vi "GV_Legend_DrawMove.vi"(2 "Legend":T1, 5 "Select":bool, 8 "Origin":cluster{"x":i16, "y":i16}) -> (7 "Image":picture)   [LabVIEW 2020, in "Sgraph_lib_V1.lvlib" / "Gviewer.lvclass"]
doc: "Andre Koelewijn, 25 April 2021,\n\nDraw arrows around the Legend to indicate the 'Legend-Move' grip.\nThe move action is then to be initiated by pressing the mouse button or the (s)elect button."
uses:
  Gviewer.lvclass
  controls/LegendSet.ctl
  <vilib>/Utility/miscctls.llb/LVPositionTypeDef.ctl
  <vilib>/Utility/miscctls.llb/LVBoundsTypeDef.ctl
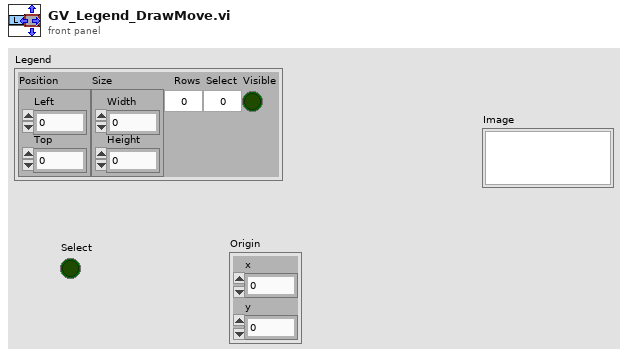
[diagram p1: front panel]
types:
  T1 = typedef "Sgraph_lib_V1.lvlib/Gviewer.lvclass/LegendSet.ctl" = cluster{"Position":T2, "Size":T3, "Rows":u32, "Select":i32, "Visible":bool}
  T2 = typedef "LVPositionTypeDef.ctl" = cluster{"Left":i32, "Top":i32}
  T3 = typedef "LVBoundsTypeDef.ctl" = cluster{"Width":u32, "Height":u32}
  T4 = cluster{"Width":u16, "Style":enum32{"Solid", "Dash", "Dot", "DashDot", "DashDotDot"}}
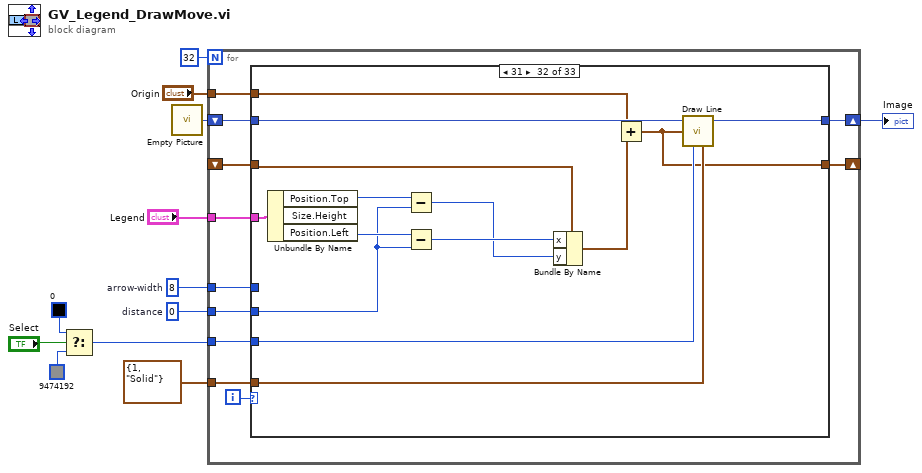
[diagram p0: block diagram]
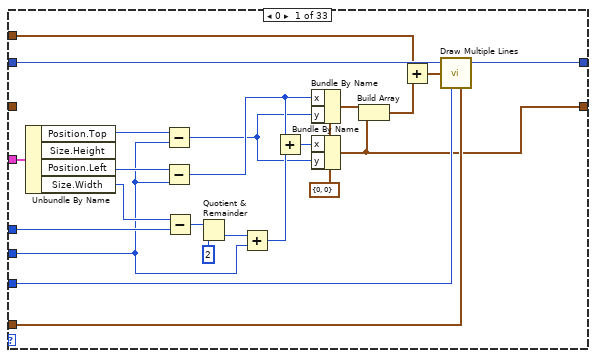
[diagram p2: hidden frame]
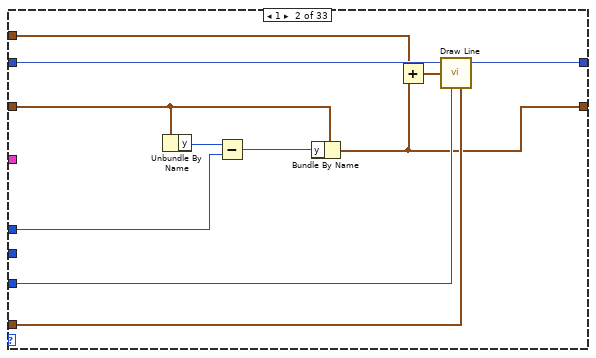
[diagram p3: hidden frame]
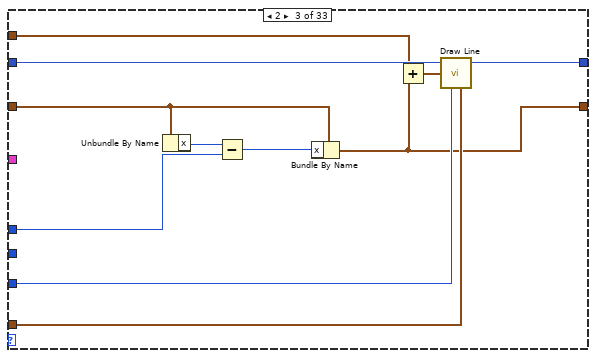
[diagram p4: hidden frame]
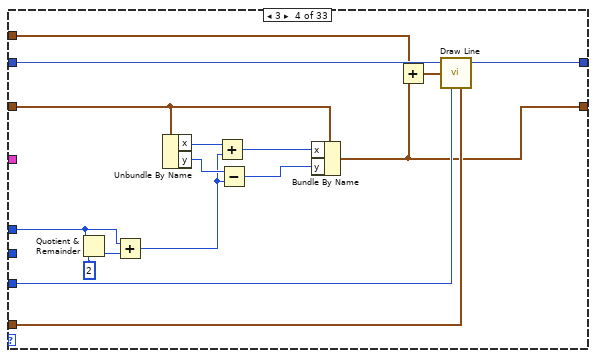
[diagram p5: hidden frame]
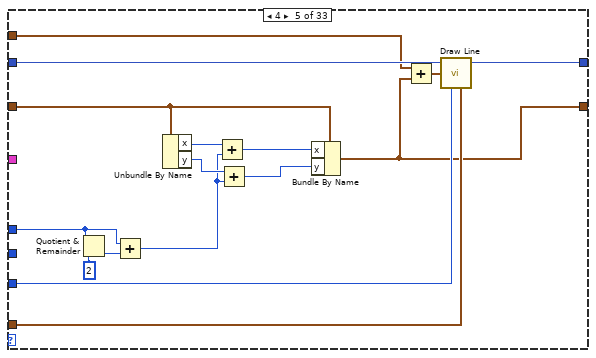
[diagram p6: hidden frame]
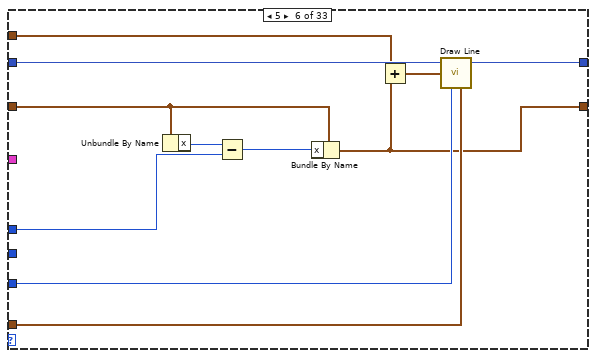
[diagram p7: hidden frame]
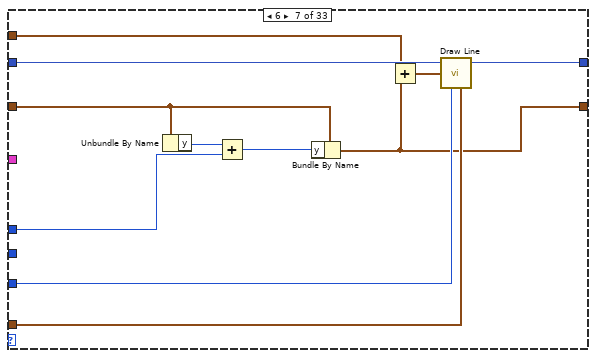
[diagram p8: hidden frame]
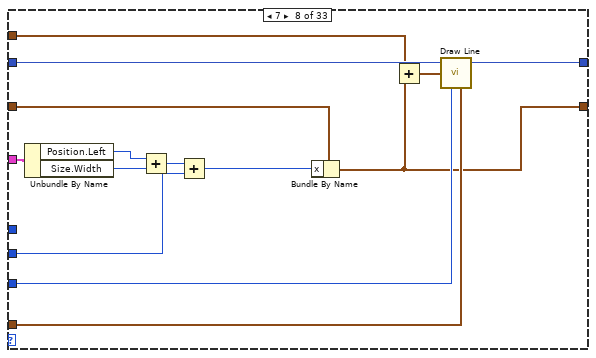
[diagram p9: hidden frame]
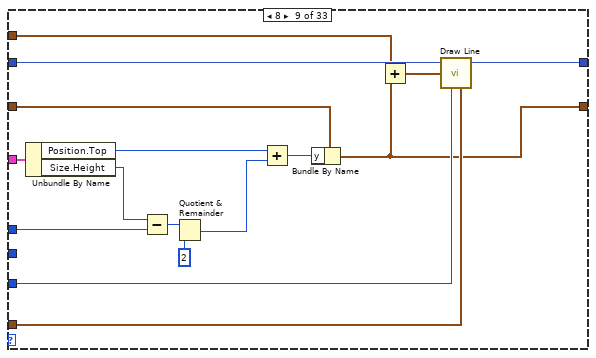
[diagram p10: hidden frame]
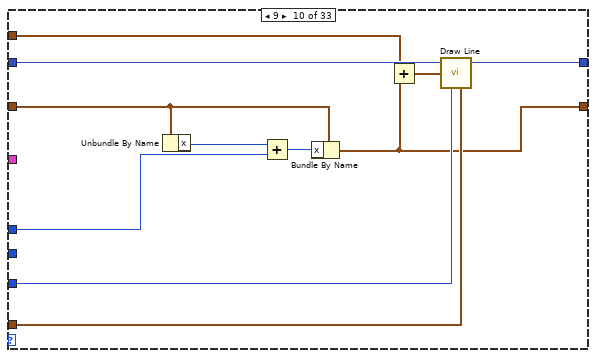
[diagram p11: hidden frame]
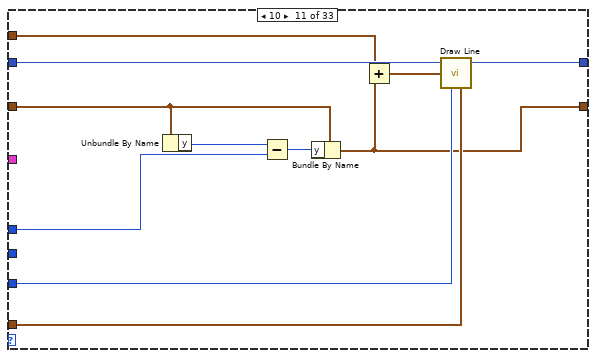
[diagram p12: hidden frame]
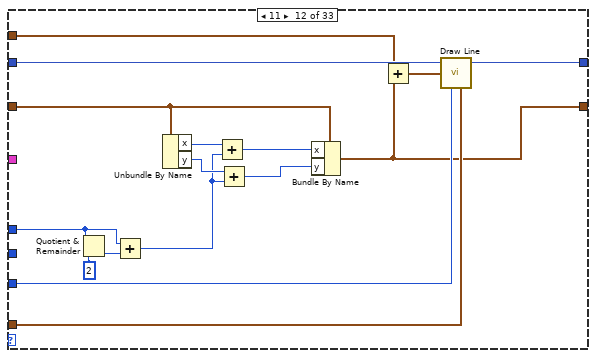
[diagram p13: hidden frame]
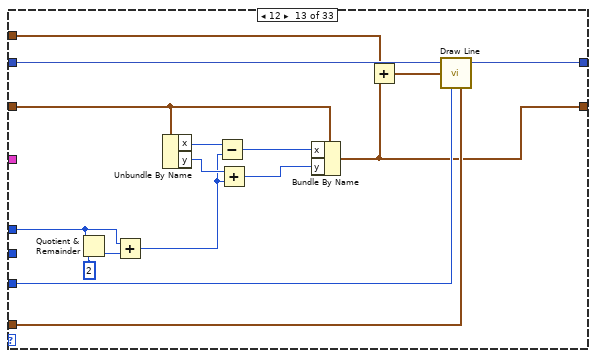
[diagram p14: hidden frame]
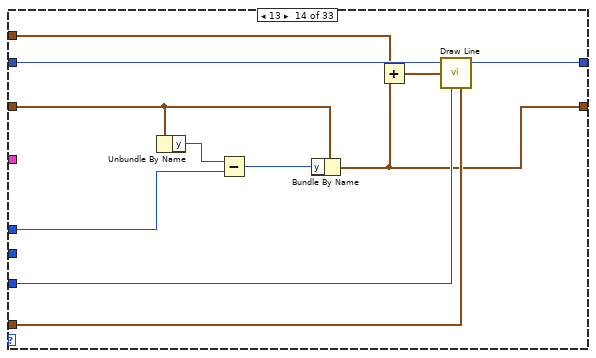
[diagram p15: hidden frame]
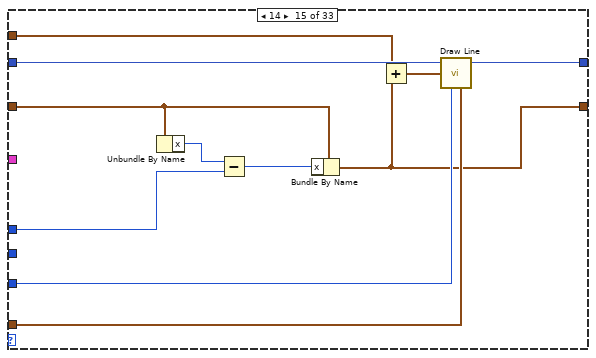
[diagram p16: hidden frame]
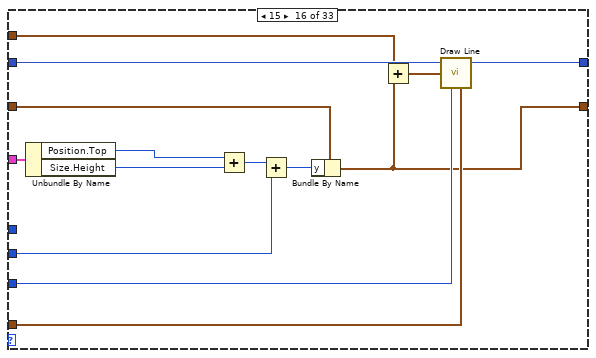
[diagram p17: hidden frame]
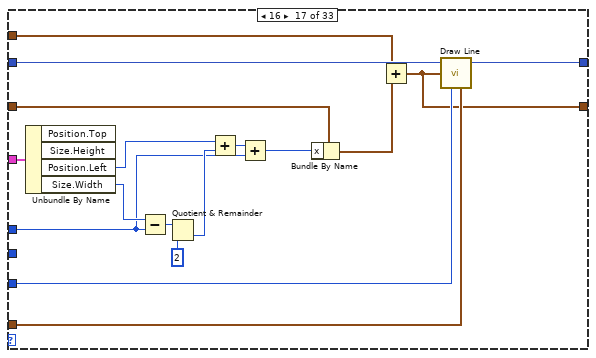
[diagram p18: hidden frame]
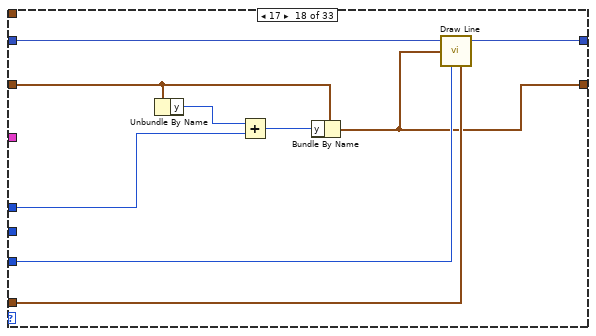
[diagram p19: hidden frame]
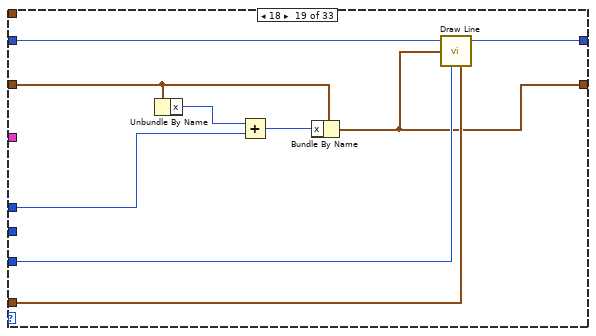
[diagram p20: hidden frame]
diagram:
  w6 = i16 8  # arrow-width
  w7 = i16 0  # distance
  n1 = Select(t=u32 0, s="Select", f=u32 9474192) -> (s? t:f=w1:u32)
  n2 = call "Empty Picture"() -> ("empty picture"=w12:picture)
  n3 = for {
    N: 32 -> [_]
    shift-right: [w20] -> w9
    shift-left: w12 -> [w21]
    tunnel: "Legend" -> [w22]
    tunnel: w1 -> [w19]
    tunnel: T4 {"Width"=1, "Style"=enum."Solid"} ("pen") -> [w18]
    tunnel: w7 -> [w17]
    tunnel: w6 -> [w16]
    shift-right: [w15] -> _
    shift-left: _ -> [w14]
    tunnel: "Origin" -> [w13]
    i -> [w23]
    n4 = case shown="31" w23 {
      tunnel: w22 -> [w42 _ _ _ _ _ _ w132 w148 _ _ _ _ _ _ w238 w255 _ _ _ _ _ _ w335 w351 _ _ _ _ _ _ w429 _]
      tunnel: w21 -> [w46 w57 w68 w84 w100 w111 w122 w136 w152 w163 w174 w190 w206 w217 w228 w242 w259 w268 w277 w291 w305 w314 w323 w339 w355 w364 w373 w387 w401 w410 w419 w433 w435]
      tunnel: [w45 w56 w67 w83 w99 w110 w121 w135 w151 w162 w173 w189 w205 w216 w227 w241 w258 w267 w276 w290 w304 w313 w322 w338 w354 w363 w372 w386 w400 w409 w418 w432 w435] -> w20
      tunnel: w19 -> [w44 w55 w66 w82 w98 w109 w120 w134 w150 w161 w172 w188 w204 w215 w226 w240 w257 w266 w275 w289 w303 w312 w321 w337 w353 w362 w371 w385 w399 w408 w417 w431 _]
      tunnel: w18 -> [w43 w54 w65 w81 w97 w108 w119 w133 w149 w160 w171 w187 w203 w214 w225 w239 w256 w265 w274 w288 w302 w311 w320 w336 w352 w361 w370 w384 w398 w407 w416 w430 _]
      tunnel: w17 -> [w30 _ _ _ _ _ _ w127 _ _ _ _ _ _ _ w231 _ _ _ _ _ _ _ w325 w341 _ _ _ _ _ _ w425 _]
      tunnel: w16 -> [w34 w50 w61 w74 w90 w104 w115 _ w143 w156 w167 w180 w196 w210 w221 _ w247 w263 w272 w280 w294 w309 w318 _ w346 w359 w368 w376 w390 w402 w411 _ _]
      tunnel: [w31 w48 w60 w70 w87 w102 w113 w124 w139 w154 w165 w176 w192 w208 w219 w233 w243 w264 w273 w287 w301 w310 w319 w329 w349 w360 w369 w383 w397 w406 w415 w421 w434] -> w15
      tunnel: w14 -> [_ w53 w64 w80 w96 w107 w118 w131 w146 w159 w170 w186 w202 w213 w224 w237 w252 w261 w270 w286 w300 w307 w316 w334 w345 w357 w366 w382 w396 w405 w414 w420 w434]
      tunnel: w13 -> [w25 w49 w59 w71 w85 w103 w114 w125 w140 w155 w166 w177 w193 w209 w220 w234 w245 _ _ _ _ _ _ w331 _ _ _ _ _ _ _ w423 _]
      frame 0 {
        w40 = cluster{"x":i16, "y":i16} {"x"=0, "y"=0}
        n5 = Unbundle By Name(w42) -> ("Position.Top"=w38:i32, "Position.Left"=w41:i32, "Size.Width"=w35:u32)  [unwired: 1 out]
        n6 = Subtract(x=w38, y=w30) -> (x-y=w27:i32)
        n7 = Subtract(x=w41, y=w30) -> (x-y=w37:i32)
        n8 = Subtract(x=w35, y=w34) -> (x-y=w33:u32)
        n9 = Quotient & Remainder(x=w33, y=u32 2) -> (floor(x/y)=w29:u32)  [unwired: 1 out]
        n10 = Add(x=w29, y=w30) -> (x+y=w28:u32)
        n11 = Add(x=w37, y=w28) -> (x+y=w36:u32)
        n12 = Bundle By Name(cluster=w40, "x"=w37, "y"=w27) -> (w39:cluster{"x":i16, "y":i16})
        n13 = Bundle By Name(cluster=w40, "x"=w36, "y"=w27) -> (w31:cluster{"x":i16, "y":i16})
        n14 = Build Array(w39, w31) -> (w26:cluster{"x":i16, "y":i16}[])
        n15 = Add(x=w25, y=w26) -> (x+y=w24:cluster{"x":i16, "y":i16}[])
        n16 = call <vilib>:"Draw Multiple Lines.vi"("picture"=w46, "line endpoints"=w24, "color(black)"=w44, "pen"=w43) -> ("new picture"=w45:picture)  [unwired: 5 in]
      }
      frame 1 {
        n17 = Unbundle By Name(w53) -> ("y"=w52:i16)
        n18 = Subtract(x=w52, y=w50) -> (x-y=w51:i16)
        n19 = Bundle By Name(cluster=w53, "y"=w51) -> (w48:cluster{"x":i16, "y":i16})
        n20 = Add(x=w49, y=w48) -> (x+y=w47:cluster{"x":i16, "y":i16})
        n21 = call <vilib>:"Draw Line.vi"("picture"=w57, "end point"=w47, "color(black)"=w55, "pen"=w54) -> ("new picture"=w56:picture)  [unwired: 5 in]
      }
      frame 2 {
        n22 = Unbundle By Name(w64) -> ("x"=w63:i16)
        n23 = Subtract(x=w63, y=w61) -> (x-y=w62:i16)
        n24 = Bundle By Name(cluster=w64, "x"=w62) -> (w60:cluster{"x":i16, "y":i16})
        n25 = Add(x=w59, y=w60) -> (x+y=w58:cluster{"x":i16, "y":i16})
        n26 = call <vilib>:"Draw Line.vi"("picture"=w68, "end point"=w58, "color(black)"=w66, "pen"=w65) -> ("new picture"=w67:picture)  [unwired: 5 in]
      }
      frame 3 {
        n27 = Quotient & Remainder(x=w74, y=u32 2) -> (floor(x/y)=w75:u32)  [unwired: 1 out]
        n28 = Add(x=w74, y=w75) -> (x+y=w72:u32)
        n29 = Unbundle By Name(w80) -> ("x"=w79:i16, "y"=w78:i16)
        n30 = Add(x=w79, y=w72) -> (x+y=w73:u32)
        n31 = Subtract(x=w78, y=w72) -> (x-y=w77:u32)
        n32 = Bundle By Name(cluster=w80, "x"=w73, "y"=w77) -> (w70:cluster{"x":i16, "y":i16})
        n33 = Add(x=w71, y=w70) -> (x+y=w69:cluster{"x":i16, "y":i16})
        n34 = call <vilib>:"Draw Line.vi"("picture"=w84, "end point"=w69, "color(black)"=w82, "pen"=w81) -> ("new picture"=w83:picture)  [unwired: 5 in]
      }
      frame 4 {
        n35 = Quotient & Remainder(x=w90, y=u32 2) -> (floor(x/y)=w91:u32)  [unwired: 1 out]
        n36 = Add(x=w90, y=w91) -> (x+y=w88:u32)
        n37 = Unbundle By Name(w96) -> ("x"=w95:i16, "y"=w94:i16)
        n38 = Add(x=w95, y=w88) -> (x+y=w89:u32)
        n39 = Add(x=w94, y=w88) -> (x+y=w93:u32)
        n40 = Bundle By Name(cluster=w96, "x"=w89, "y"=w93) -> (w87:cluster{"x":i16, "y":i16})
        n41 = Add(x=w85, y=w87) -> (x+y=w86:cluster{"x":i16, "y":i16})
        n42 = call <vilib>:"Draw Line.vi"("picture"=w100, "end point"=w86, "color(black)"=w98, "pen"=w97) -> ("new picture"=w99:picture)  [unwired: 5 in]
      }
      frame 5 {
        n43 = Unbundle By Name(w107) -> ("x"=w106:i16)
        n44 = Subtract(x=w106, y=w104) -> (x-y=w105:i16)
        n45 = Bundle By Name(cluster=w107, "x"=w105) -> (w102:cluster{"x":i16, "y":i16})
        n46 = Add(x=w103, y=w102) -> (x+y=w101:cluster{"x":i16, "y":i16})
        n47 = call <vilib>:"Draw Line.vi"("picture"=w111, "end point"=w101, "color(black)"=w109, "pen"=w108) -> ("new picture"=w110:picture)  [unwired: 5 in]
      }
      frame 6 {
        n48 = Unbundle By Name(w118) -> ("y"=w117:i16)
        n49 = Add(x=w117, y=w115) -> (x+y=w116:i16)
        n50 = Bundle By Name(cluster=w118, "y"=w116) -> (w113:cluster{"x":i16, "y":i16})
        n51 = Add(x=w114, y=w113) -> (x+y=w112:cluster{"x":i16, "y":i16})
        n52 = call <vilib>:"Draw Line.vi"("picture"=w122, "end point"=w112, "color(black)"=w120, "pen"=w119) -> ("new picture"=w121:picture)  [unwired: 5 in]
      }
      frame 7 {
        n53 = Unbundle By Name(w132) -> ("Position.Left"=w129:i32, "Size.Width"=w130:u32)
        n54 = Add(x=w129, y=w130) -> (x+y=w128:u32)
        n55 = Add(x=w128, y=w127) -> (x+y=w126:u32)
        n56 = Bundle By Name(cluster=w131, "x"=w126) -> (w124:cluster{"x":i16, "y":i16})
        n57 = Add(x=w125, y=w124) -> (x+y=w123:cluster{"x":i16, "y":i16})
        n58 = call <vilib>:"Draw Line.vi"("picture"=w136, "end point"=w123, "color(black)"=w134, "pen"=w133) -> ("new picture"=w135:picture)  [unwired: 5 in]
      }
      frame 8 {
        n59 = Unbundle By Name(w148) -> ("Position.Top"=w137:i32, "Size.Height"=w141:u32)
        n60 = Subtract(x=w141, y=w143) -> (x-y=w145:u32)
        n61 = Quotient & Remainder(x=w145, y=u32 2) -> (floor(x/y)=w142:u32)  [unwired: 1 out]
        n62 = Add(x=w137, y=w142) -> (x+y=w144:u32)
        n63 = Bundle By Name(cluster=w146, "y"=w144) -> (w139:cluster{"x":i16, "y":i16})
        n64 = Add(x=w140, y=w139) -> (x+y=w138:cluster{"x":i16, "y":i16})
        n65 = call <vilib>:"Draw Line.vi"("picture"=w152, "end point"=w138, "color(black)"=w150, "pen"=w149) -> ("new picture"=w151:picture)  [unwired: 5 in]
      }
      frame 9 {
        n66 = Unbundle By Name(w159) -> ("x"=w158:i16)
        n67 = Add(x=w158, y=w156) -> (x+y=w157:i16)
        n68 = Bundle By Name(cluster=w159, "x"=w157) -> (w154:cluster{"x":i16, "y":i16})
        n69 = Add(x=w155, y=w154) -> (x+y=w153:cluster{"x":i16, "y":i16})
        n70 = call <vilib>:"Draw Line.vi"("picture"=w163, "end point"=w153, "color(black)"=w161, "pen"=w160) -> ("new picture"=w162:picture)  [unwired: 5 in]
      }
      frame 10 {
        n71 = Unbundle By Name(w170) -> ("y"=w169:i16)
        n72 = Subtract(x=w169, y=w167) -> (x-y=w168:i16)
        n73 = Bundle By Name(cluster=w170, "y"=w168) -> (w165:cluster{"x":i16, "y":i16})
        n74 = Add(x=w166, y=w165) -> (x+y=w164:cluster{"x":i16, "y":i16})
        n75 = call <vilib>:"Draw Line.vi"("picture"=w174, "end point"=w164, "color(black)"=w172, "pen"=w171) -> ("new picture"=w173:picture)  [unwired: 5 in]
      }
      frame 11 {
        n76 = Quotient & Remainder(x=w180, y=u32 2) -> (floor(x/y)=w181:u32)  [unwired: 1 out]
        n77 = Add(x=w180, y=w181) -> (x+y=w178:u32)
        n78 = Unbundle By Name(w186) -> ("x"=w185:i16, "y"=w184:i16)
        n79 = Add(x=w185, y=w178) -> (x+y=w179:u32)
        n80 = Add(x=w184, y=w178) -> (x+y=w183:u32)
        n81 = Bundle By Name(cluster=w186, "x"=w179, "y"=w183) -> (w176:cluster{"x":i16, "y":i16})
        n82 = Add(x=w177, y=w176) -> (x+y=w175:cluster{"x":i16, "y":i16})
        n83 = call <vilib>:"Draw Line.vi"("picture"=w190, "end point"=w175, "color(black)"=w188, "pen"=w187) -> ("new picture"=w189:picture)  [unwired: 5 in]
      }
      frame 12 {
        n84 = Quotient & Remainder(x=w196, y=u32 2) -> (floor(x/y)=w197:u32)  [unwired: 1 out]
        n85 = Add(x=w196, y=w197) -> (x+y=w194:u32)
        n86 = Unbundle By Name(w202) -> ("x"=w201:i16, "y"=w200:i16)
        n87 = Subtract(x=w201, y=w194) -> (x-y=w195:u32)
        n88 = Add(x=w200, y=w194) -> (x+y=w199:u32)
        n89 = Bundle By Name(cluster=w202, "x"=w195, "y"=w199) -> (w192:cluster{"x":i16, "y":i16})
        n90 = Add(x=w193, y=w192) -> (x+y=w191:cluster{"x":i16, "y":i16})
        n91 = call <vilib>:"Draw Line.vi"("picture"=w206, "end point"=w191, "color(black)"=w204, "pen"=w203) -> ("new picture"=w205:picture)  [unwired: 5 in]
      }
      frame 13 {
        n92 = Unbundle By Name(w213) -> ("y"=w212:i16)
        n93 = Subtract(x=w212, y=w210) -> (x-y=w211:i16)
        n94 = Bundle By Name(cluster=w213, "y"=w211) -> (w208:cluster{"x":i16, "y":i16})
        n95 = Add(x=w209, y=w208) -> (x+y=w207:cluster{"x":i16, "y":i16})
        n96 = call <vilib>:"Draw Line.vi"("picture"=w217, "end point"=w207, "color(black)"=w215, "pen"=w214) -> ("new picture"=w216:picture)  [unwired: 5 in]
      }
      frame 14 {
        n97 = Unbundle By Name(w224) -> ("x"=w223:i16)
        n98 = Subtract(x=w223, y=w221) -> (x-y=w222:i16)
        n99 = Bundle By Name(cluster=w224, "x"=w222) -> (w219:cluster{"x":i16, "y":i16})
        n100 = Add(x=w220, y=w219) -> (x+y=w218:cluster{"x":i16, "y":i16})
        n101 = call <vilib>:"Draw Line.vi"("picture"=w228, "end point"=w218, "color(black)"=w226, "pen"=w225) -> ("new picture"=w227:picture)  [unwired: 5 in]
      }
      frame 15 {
        n102 = Unbundle By Name(w238) -> ("Position.Top"=w236:i32, "Size.Height"=w235:u32)
        n103 = Add(x=w236, y=w235) -> (x+y=w230:u32)
        n104 = Add(x=w230, y=w231) -> (x+y=w229:u32)
        n105 = Bundle By Name(cluster=w237, "y"=w229) -> (w233:cluster{"x":i16, "y":i16})
        n106 = Add(x=w234, y=w233) -> (x+y=w232:cluster{"x":i16, "y":i16})
        n107 = call <vilib>:"Draw Line.vi"("picture"=w242, "end point"=w232, "color(black)"=w240, "pen"=w239) -> ("new picture"=w241:picture)  [unwired: 5 in]
      }
      frame 16 {
        n108 = Unbundle By Name(w255) -> ("Position.Left"=w250:i32, "Size.Width"=w254:u32)  [unwired: 2 out]
        n109 = Subtract(x=w254, y=w247) -> (x-y=w251:u32)
        n110 = Quotient & Remainder(x=w251, y=u32 2) -> (floor(x/y)=w249:u32)  [unwired: 1 out]
        n111 = Add(x=w250, y=w249) -> (x+y=w248:u32)
        n112 = Add(x=w248, y=w247) -> (x+y=w246:u32)
        n113 = Bundle By Name(cluster=w252, "x"=w246) -> (w244:cluster{"x":i16, "y":i16})
        n114 = Add(x=w245, y=w244) -> (x+y=w243:cluster{"x":i16, "y":i16})
        n115 = call <vilib>:"Draw Line.vi"("picture"=w259, "end point"=w243, "color(black)"=w257, "pen"=w256) -> ("new picture"=w258:picture)  [unwired: 5 in]
      }
      frame 17 {
        n116 = Unbundle By Name(w261) -> ("y"=w260:i16)
        n117 = Add(x=w260, y=w263) -> (x+y=w262:i16)
        n118 = Bundle By Name(cluster=w261, "y"=w262) -> (w264:cluster{"x":i16, "y":i16})
        n119 = call <vilib>:"Draw Line.vi"("picture"=w268, "end point"=w264, "color(black)"=w266, "pen"=w265) -> ("new picture"=w267:picture)  [unwired: 5 in]
      }
      frame 18 {
        n120 = Unbundle By Name(w270) -> ("x"=w269:i16)
        n121 = Add(x=w269, y=w272) -> (x+y=w271:i16)
        n122 = Bundle By Name(cluster=w270, "x"=w271) -> (w273:cluster{"x":i16, "y":i16})
        n123 = call <vilib>:"Draw Line.vi"("picture"=w277, "end point"=w273, "color(black)"=w275, "pen"=w274) -> ("new picture"=w276:picture)  [unwired: 5 in]
      }
      frame 19 {
        n124 = Quotient & Remainder(x=w280, y=u32 2) -> (floor(x/y)=w281:u32)  [unwired: 1 out]
        n125 = Add(x=w280, y=w281) -> (x+y=w278:u32)
        n126 = Unbundle By Name(w286) -> ("x"=w285:i16, "y"=w284:i16)
        n127 = Subtract(x=w285, y=w278) -> (x-y=w279:u32)
        n128 = Add(x=w284, y=w278) -> (x+y=w283:u32)
        n129 = Bundle By Name(cluster=w286, "x"=w279, "y"=w283) -> (w287:cluster{"x":i16, "y":i16})
        n130 = call <vilib>:"Draw Line.vi"("picture"=w291, "end point"=w287, "color(black)"=w289, "pen"=w288) -> ("new picture"=w290:picture)  [unwired: 5 in]
      }
      frame 20 {
        n131 = Quotient & Remainder(x=w294, y=u32 2) -> (floor(x/y)=w295:u32)  [unwired: 1 out]
        n132 = Add(x=w294, y=w295) -> (x+y=w292:u32)
        n133 = Unbundle By Name(w300) -> ("x"=w299:i16, "y"=w298:i16)
        n134 = Subtract(x=w299, y=w292) -> (x-y=w293:u32)
        n135 = Subtract(x=w298, y=w292) -> (x-y=w297:u32)
        n136 = Bundle By Name(cluster=w300, "x"=w293, "y"=w297) -> (w301:cluster{"x":i16, "y":i16})
        n137 = call <vilib>:"Draw Line.vi"("picture"=w305, "end point"=w301, "color(black)"=w303, "pen"=w302) -> ("new picture"=w304:picture)  [unwired: 5 in]
      }
      frame 21 {
        n138 = Unbundle By Name(w307) -> ("x"=w306:i16)
        n139 = Add(x=w306, y=w309) -> (x+y=w308:i16)
        n140 = Bundle By Name(cluster=w307, "x"=w308) -> (w310:cluster{"x":i16, "y":i16})
        n141 = call <vilib>:"Draw Line.vi"("picture"=w314, "end point"=w310, "color(black)"=w312, "pen"=w311) -> ("new picture"=w313:picture)  [unwired: 5 in]
      }
      frame 22 {
        n142 = Unbundle By Name(w316) -> ("y"=w315:i16)
        n143 = Subtract(x=w315, y=w318) -> (x-y=w317:i16)
        n144 = Bundle By Name(cluster=w316, "y"=w317) -> (w319:cluster{"x":i16, "y":i16})
        n145 = call <vilib>:"Draw Line.vi"("picture"=w323, "end point"=w319, "color(black)"=w321, "pen"=w320) -> ("new picture"=w322:picture)  [unwired: 5 in]
      }
      frame 23 {
        n146 = Unbundle By Name(w335) -> ("Position.Top"=w328:i32, "Size.Height"=w327:u32, "Position.Left"=w333:i32)
        n147 = Add(x=w328, y=w327) -> (x+y=w326:u32)
        n148 = Subtract(x=w333, y=w325) -> (x-y=w332:i32)
        n149 = Add(x=w326, y=w325) -> (x+y=w324:u32)
        n150 = Bundle By Name(cluster=w334, "y"=w324, "x"=w332) -> (w330:cluster{"x":i16, "y":i16})
        n151 = Add(x=w331, y=w330) -> (x+y=w329:cluster{"x":i16, "y":i16})
        n152 = call <vilib>:"Draw Line.vi"("picture"=w339, "end point"=w329, "color(black)"=w337, "pen"=w336) -> ("new picture"=w338:picture)  [unwired: 5 in]
      }
      frame 24 {
        n153 = Unbundle By Name(w351) -> ("Size.Height"=w347:u32)  [unwired: 3 out]
        n154 = Subtract(x=w347, y=w346) -> (x-y=w348:u32)
        n155 = Quotient & Remainder(x=w348, y=u32 2) -> (floor(x/y)=w342:u32)  [unwired: 1 out]
        n156 = Unbundle By Name(w345) -> ("y"=w344:i16)
        n157 = Add(x=w342, y=w341) -> (x+y=w340:u32)
        n158 = Subtract(x=w344, y=w340) -> (x-y=w343:u32)
        n159 = Bundle By Name(cluster=w345, "y"=w343) -> (w349:cluster{"x":i16, "y":i16})
        n160 = call <vilib>:"Draw Line.vi"("picture"=w355, "end point"=w349, "color(black)"=w353, "pen"=w352) -> ("new picture"=w354:picture)  [unwired: 5 in]
      }
      frame 25 {
        n161 = Unbundle By Name(w357) -> ("x"=w356:i16)
        n162 = Subtract(x=w356, y=w359) -> (x-y=w358:i16)
        n163 = Bundle By Name(cluster=w357, "x"=w358) -> (w360:cluster{"x":i16, "y":i16})
        n164 = call <vilib>:"Draw Line.vi"("picture"=w364, "end point"=w360, "color(black)"=w362, "pen"=w361) -> ("new picture"=w363:picture)  [unwired: 5 in]
      }
      frame 26 {
        n165 = Unbundle By Name(w366) -> ("y"=w365:i16)
        n166 = Add(x=w365, y=w368) -> (x+y=w367:i16)
        n167 = Bundle By Name(cluster=w366, "y"=w367) -> (w369:cluster{"x":i16, "y":i16})
        n168 = call <vilib>:"Draw Line.vi"("picture"=w373, "end point"=w369, "color(black)"=w371, "pen"=w370) -> ("new picture"=w372:picture)  [unwired: 5 in]
      }
      frame 27 {
        n169 = Quotient & Remainder(x=w376, y=u32 2) -> (floor(x/y)=w377:u32)  [unwired: 1 out]
        n170 = Add(x=w376, y=w377) -> (x+y=w374:u32)
        n171 = Unbundle By Name(w382) -> ("x"=w381:i16, "y"=w380:i16)
        n172 = Subtract(x=w381, y=w374) -> (x-y=w375:u32)
        n173 = Subtract(x=w380, y=w374) -> (x-y=w379:u32)
        n174 = Bundle By Name(cluster=w382, "x"=w375, "y"=w379) -> (w383:cluster{"x":i16, "y":i16})
        n175 = call <vilib>:"Draw Line.vi"("picture"=w387, "end point"=w383, "color(black)"=w385, "pen"=w384) -> ("new picture"=w386:picture)  [unwired: 5 in]
      }
      frame 28 {
        n176 = Quotient & Remainder(x=w390, y=u32 2) -> (floor(x/y)=w391:u32)  [unwired: 1 out]
        n177 = Add(x=w390, y=w391) -> (x+y=w388:u32)
        n178 = Unbundle By Name(w396) -> ("x"=w395:i16, "y"=w394:i16)
        n179 = Add(x=w395, y=w388) -> (x+y=w389:u32)
        n180 = Subtract(x=w394, y=w388) -> (x-y=w393:u32)
        n181 = Bundle By Name(cluster=w396, "x"=w389, "y"=w393) -> (w397:cluster{"x":i16, "y":i16})
        n182 = call <vilib>:"Draw Line.vi"("picture"=w401, "end point"=w397, "color(black)"=w399, "pen"=w398) -> ("new picture"=w400:picture)  [unwired: 5 in]
      }
      frame 29 {
        n183 = Unbundle By Name(w405) -> ("y"=w404:i16)
        n184 = Add(x=w404, y=w402) -> (x+y=w403:i16)
        n185 = Bundle By Name(cluster=w405, "y"=w403) -> (w406:cluster{"x":i16, "y":i16})
        n186 = call <vilib>:"Draw Line.vi"("picture"=w410, "end point"=w406, "color(black)"=w408, "pen"=w407) -> ("new picture"=w409:picture)  [unwired: 5 in]
      }
      frame 30 {
        n187 = Unbundle By Name(w414) -> ("x"=w413:i16)
        n188 = Add(x=w413, y=w411) -> (x+y=w412:i16)
        n189 = Bundle By Name(cluster=w414, "x"=w412) -> (w415:cluster{"x":i16, "y":i16})
        n190 = call <vilib>:"Draw Line.vi"("picture"=w419, "end point"=w415, "color(black)"=w417, "pen"=w416) -> ("new picture"=w418:picture)  [unwired: 5 in]
      }
      frame 31 {
        n191 = Unbundle By Name(w429) -> ("Position.Top"=w427:i32, "Position.Left"=w428:i32)  [unwired: 1 out]
        n192 = Subtract(x=w427, y=w425) -> (x-y=w424:i32)
        n193 = Subtract(x=w428, y=w425) -> (x-y=w426:i32)
        n194 = Bundle By Name(cluster=w420, "x"=w426, "y"=w424) -> (w422:cluster{"x":i16, "y":i16})
        n195 = Add(x=w423, y=w422) -> (x+y=w421:cluster{"x":i16, "y":i16})
        n196 = call <vilib>:"Draw Line.vi"("picture"=w433, "end point"=w421, "color(black)"=w431, "pen"=w430) -> ("new picture"=w432:picture)  [unwired: 5 in]
      }
      frame Default {
      }
    }
  }
  "Image" <- w9
